vi "create wheel page.vi"(1 "all rows 2":string[][](array[string])) -> ()   [LabVIEW 2016]
panel:
  out "number":i32
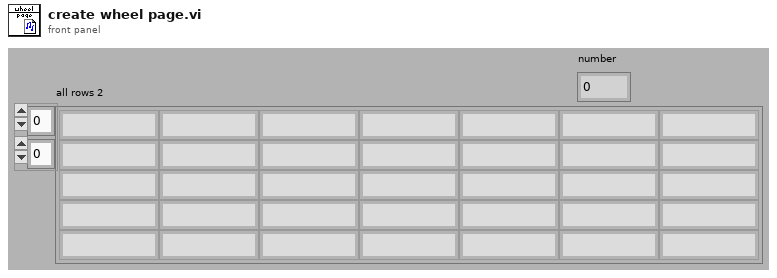
[diagram p1: front panel]
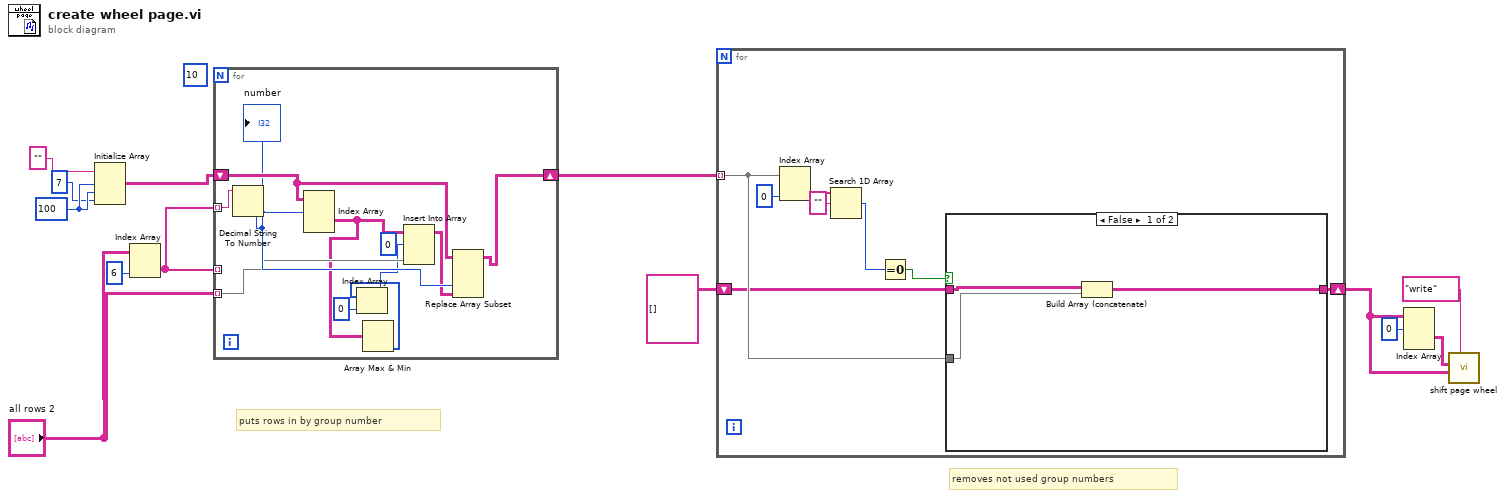
[diagram p0: block diagram]
diagram:
  (unwired) 10
  w9 = 100 ("dimension size")
  # "puts rows in by group number"
  # "removes not used group numbers"
  n1 = Initialize Array("", w9, w9, 7 ("dimension size")) -> (w7:string[][][])
  n2 = Index Array(array="all rows 2", index (col)=6 ("disabled index (col)")) -> (element=w10:string[])  [unwired: 1 in]
  n3 = for {
    tunnel: w10 -> [_] mode=indexing
    shift-right: [w18] -> w6
    shift-left: w7 -> [w22]
    tunnel: w10 -> [w23] mode=indexing
    tunnel: "all rows 2" -> [w19] mode=indexing
    (unwired) 0 ("index (row)")
    n4 = Decimal String To Number(string=w23) -> (number=w21:i32)  [unwired: 2 in, 1 out]
    "number" <- w21
    n5 = Index Array(array=w22, index (dim 0)=w21) -> (element=w16:string[][])  [unwired: 2 in]
    n6 = Array Max & Min(array=w16) -> (min index (indices)=w14:i32[])  [unwired: 3 out]
    n7 = Index Array(array=w14, index=0) -> (element=w15:i32)
    n8 = Insert Into Array(array=w16, index (row)=w15, new element=w19) -> (w20:string[][])  [unwired: 1 in]
    n9 = Replace Array Subset(array=w22, new element=w20, index (dim 0)=w21) -> (w18:string[][][])  [unwired: 2 in]
  }
  n10 = for {
    tunnel: w6 -> [w27] mode=indexing
    shift-right: [w26] -> w3
    shift-left: string[][][] [] -> [w25]
    n11 = Index Array(array=w27, index (col)=0 ("disabled index (col)")) -> (element=w24:string[])  [unwired: 1 in]
    n12 = Search 1D Array(1D array=w24, element="") -> (index of element=w29:i32)  [unwired: 1 in]
    n13 = Equal To 0?(x=w29) -> (x = 0?=w28:bool)
    n14 = case shown="False" w28 {
      tunnel: w27 -> [w32 _]
      tunnel: [w34 w35] -> w26
      tunnel: w25 -> [w33 w35]
      frame False {
        n15 = Build Array (concatenate)(w33, w32) -> (w34:string[][][])
      }
      frame True {
      }
    }
  }
  n16 = Index Array(array=w3, index (dim 0)=0 ("index (page)")) -> (element=w1:string[][])  [unwired: 2 in]
  n17 = call "shift page wheel.vi"("read write"="write", "wheel page in"=w3, "current run list in"=w1) -> ()  [unwired: 7 in, 2 out]
